vi "lorentzian transformations.vi"(7 "4 corner circle transformation":T3=enum."fix phase", 8 "lorentzian in":T2 {"bg (V)" format="%#9_9f"; "Q" format="%#9_9f"; "phi(rad)" format="%#9_9f"; "G (Hz)" format="%#9_9f"; "f (Hz)" format="%#9_9f"}, 10 "freq in":dbl, 11 "voltage in":cdb) -> (0 "lorentzian out":T2={"A (VHz)"=-1.0311345636926572, "f (Hz)"=-1.0311345636926572, "G (Hz)"=-1.0311345636926572, "phi(rad)"=-1.0311345636926572, "Q"=-1.0311345636926572, "Norm  Ampl"=-1.0311345636926572, "bg (V)"=-1.0311345636926572+0.0i, "4corners"={"z (-pi/2)"=-1.0311345636926572+0.5736824521422934i, "z(inf)"=-0.5200164984937075+1.0975277942502903i, "z (pi/2)"=-1.0311345636926572+0.5736824521422934i, "z center"=-0.5136528600391839+0.580046090596817i, "z(0)"=-0.5200164984937075+1.0975277942502903i, "radius"=-1.0311345636926572}} {"bg (V)" format="%#9_9f"; "Q" format="%#9_9f"; "phi(rad)" format="%#9_9f"; "G (Hz)" format="%#9_9f"; "f (Hz)" format="%#9_9f"}, 1 "4corners our":T1={"z (-pi/2)"=-1.0311345636926572+0.5736824521422934i, "z(inf)"=-0.5200164984937075+1.0975277942502903i, "z (pi/2)"=-1.0311345636926572+0.5736824521422934i, "z center"=-0.5136528600391839+0.580046090596817i, "z(0)"=-0.5200164984937075+1.0975277942502903i, "radius"=-1.0311345636926572}, 2 "gamma OUT":dbl, 3 "voltage out":cdb)   [LabVIEW 2018]
uses:
  four-corner circle transformation.ctl
  lorentzian.ctl
  circle corners.ctl
  Q - not nan -- real.vi
panel:
  out "freq OUT":dbl
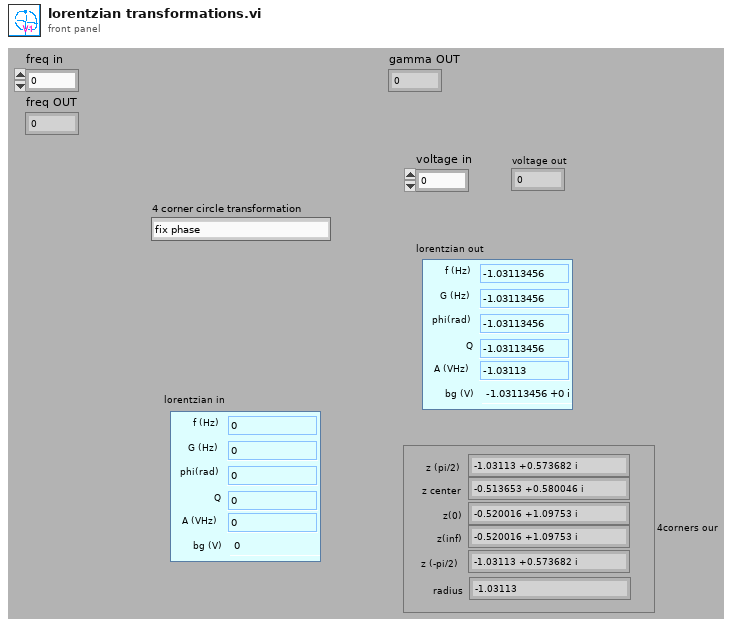
[diagram p1: front panel]
types:
  T1 = typedef "circle corners.ctl" = cluster{"z (-pi/2)":cdb, "z(inf)":cdb, "z (pi/2)":cdb, "z center":cdb, "z(0)":cdb, "radius":dbl}
  T2 = typedef "lorentzian.ctl" = cluster{"A (VHz)":dbl, "f (Hz)":dbl, "G (Hz)":dbl, "phi(rad)":dbl, "Q":dbl, "Norm  Ampl":dbl, "bg (V)":cdb, "4corners":T1}
  T3 = typedef "four-corner circle transformation.ctl" = enum16{"z(c) z(inf)", "z(c) z(zero)", "fix phase", "calculate lorentzian", "z(0) z(+-pi/2)", "shift to zcenter", "to  canonical", "get canonical phase", "get4corners", "update lorentzian -- from z0", "fake gamma normal", "fake gamma heat", "calculate complex slope"}
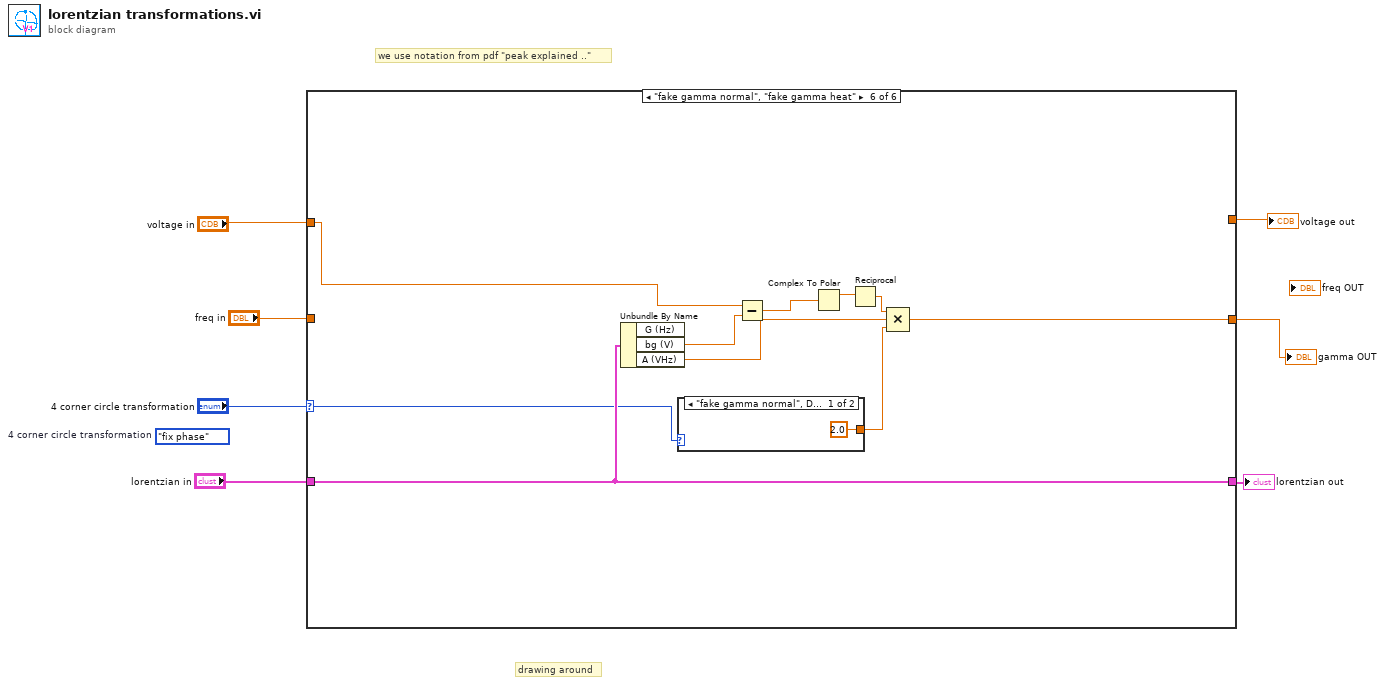
[diagram p0: block diagram]
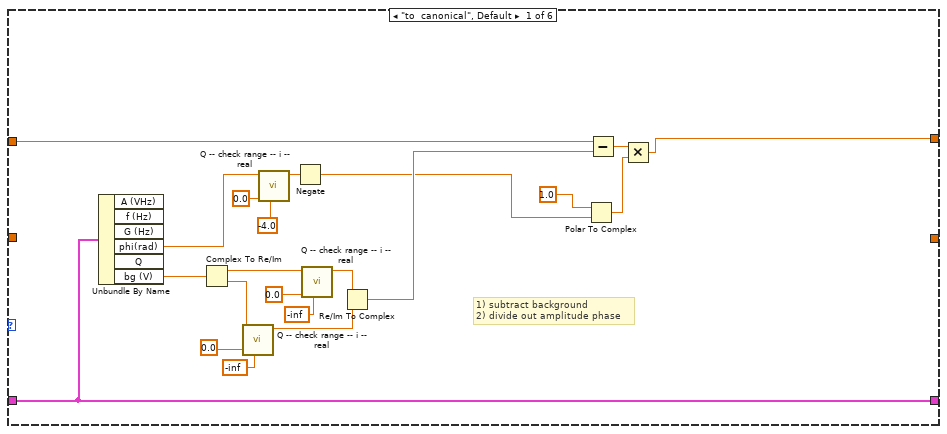
[diagram p2: hidden frame]
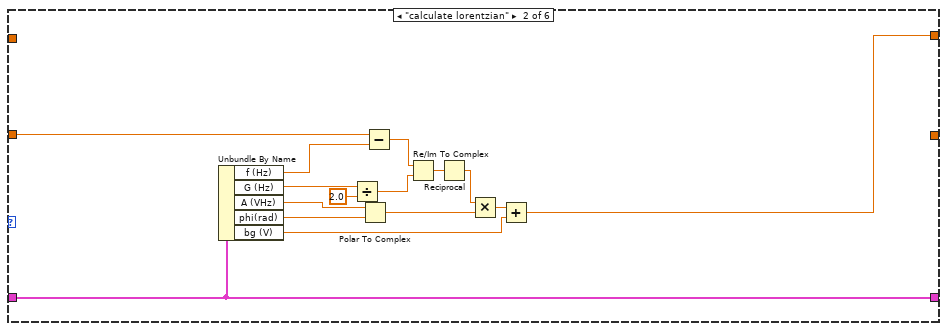
[diagram p3: hidden frame]
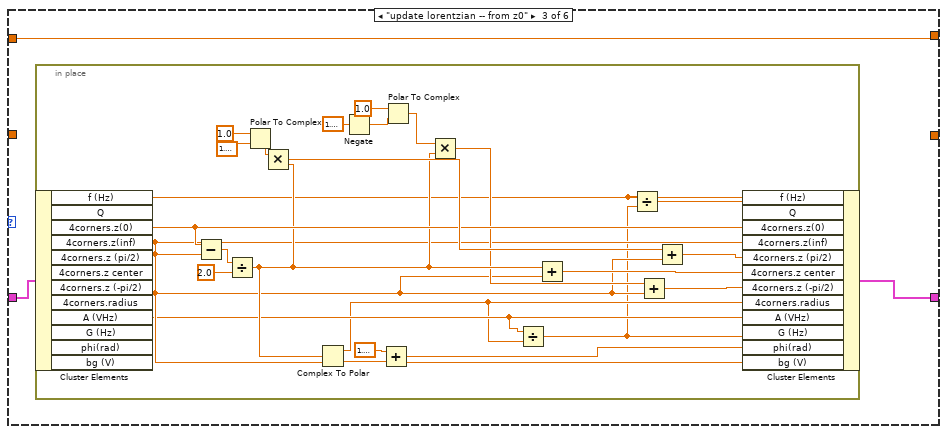
[diagram p4: hidden frame]
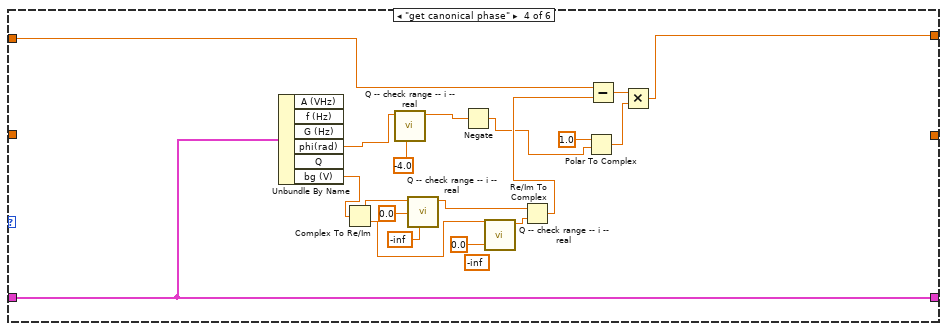
[diagram p5: hidden frame]
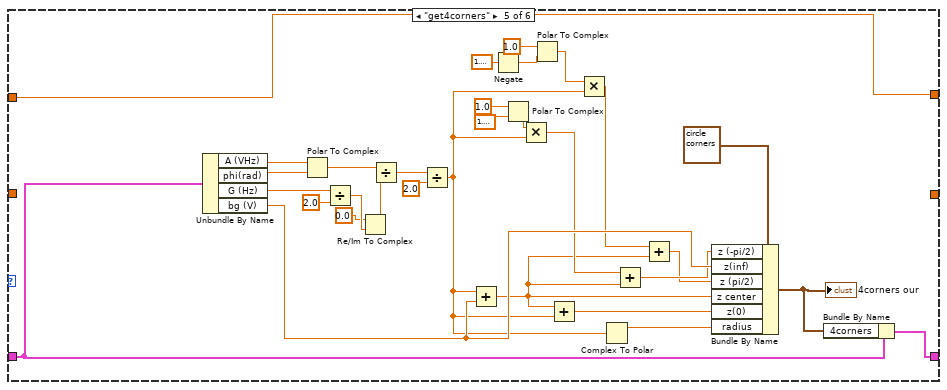
[diagram p6: hidden frame]
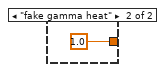
[diagram p7: hidden frame]
diagram:
  (unwired) four-corner_circle_transformation."fix phase"  # 4 corner circle transformation
  # "we use notation from pdf \"peak explained ..\""
  # "drawing around"
  n1 = case shown="\"fake gamma normal\", \"fake gamma heat\"" "4 corner circle transformation" {
    selector: "4 corner circle transformation" -> [_ _ _ _ _ w122]
    tunnel: "voltage in" -> [w11 _ w44 w73 w98 w125]
    tunnel: [w12 w43 w45 w74 w91 w124] -> w5
    tunnel: "lorentzian in" -> [w12 w43 w46 w74 w93 w124]
    tunnel: [w10 w37 w44 w72 w98 _] -> w3
    tunnel: "freq in" -> [_ w42 _ _ _ _]
    tunnel: [_ _ _ _ _ w123] -> w1
    frame "to  canonical", Default {
      # "1) subtract background\n2) divide out amplitude phase"
      n2 = Unbundle By Name(w12) -> ("phi(rad)"=w25:dbl, "bg (V)"=w23:cdb)  [unwired: 4 out]
      n3 = Complex To Re/Im(x + iy=w23) -> (x=w22:dbl, y=w20:dbl)
      n4 = call "Q -- check range -- i -- real.vi"("lower"=-inf, "default"=0.0, "number"=w20) -> ("number in range"=w17:dbl)  [unwired: 6 in, 2 out]
      n5 = call "Q -- check range -- i -- real.vi"("lower"=-4.0, "default"=0.0, "number"=w25) -> ("number in range"=w14:dbl)  [unwired: 6 in, 2 out]
      n6 = Negate(x=w14) -> (-x=w13:dbl)
      n7 = call "Q -- check range -- i -- real.vi"("lower"=-inf, "default"=0.0, "number"=w22) -> ("number in range"=w16:dbl)  [unwired: 6 in, 2 out]
      n8 = Re/Im To Complex(1:w17, 2:w16) -> (0:w15:cdb)
      n9 = Polar To Complex(1:w13, 2:1.0 ("r")) -> (0:w26:cdb)
      n10 = Subtract(x=w11, y=w15) -> (x-y=w27:cdb)
      n11 = Multiply(x=w27, y=w26) -> (x*y=w10:cdb)
    }
    frame "calculate lorentzian" {
      n12 = Unbundle By Name(w43) -> ("f (Hz)"=w30:dbl, "G (Hz)"=w29:dbl, "A (VHz)"=w31:dbl, "phi(rad)"=w41:dbl, "bg (V)"=w38:cdb)
      n13 = Divide(x=w29, y=2.0 ("x")) -> (x/y=w33:dbl)
      n14 = Polar To Complex(1:w41, 2:w31) -> (0:w40:cdb)
      n15 = Subtract(x=w42, y=w30) -> (x-y=w35:dbl)
      n16 = Re/Im To Complex(1:w33, 2:w35) -> (0:w32:cdb)
      n17 = Reciprocal(x=w32) -> (1/x=w36:cdb)
      n18 = Multiply(x=w36, y=w40) -> (x*y=w39:cdb)
      n19 = Add(x=w39, y=w38) -> (x+y=w37:cdb)
    }
    frame "update lorentzian -- from z0" {
      n20 = in-place {
        n21 = in-place-cluster #1(w46) -> ("f (Hz)"=w49:dbl, "4corners.z(0)"=w56:cdb, "4corners.z(inf)"=w52:cdb, "A (VHz)"=w51:dbl)  [unwired: 8 out]
        n22 = Subtract(x=w56, y=w52) -> (x-y=w67:cdb)
        n23 = Divide(x=w67, y=2.0) -> (x/y=w55:cdb)
        n24 = Polar To Complex(1:1.5707963267948966, 2:1.0 ("r")) -> (0:w60:cdb)
        n25 = Multiply(x=w60, y=w55) -> (x*y=w58:cdb)
        n26 = Complex To Polar(r * e^(i*theta)=w55) -> (r=w50:dbl, theta=w70:dbl)
        n27 = Negate(x=1.5707963267948966) -> (-x=w61:dbl)
        n28 = Add(x=1.5707963267948966, y=w70) -> (x+y=w69:dbl)
        n29 = Polar To Complex(1:w61, 2:1.0 ("r")) -> (0:w59:cdb)
        n30 = Multiply(x=w59, y=w55) -> (x*y=w54:cdb)
        n31 = Divide(x=w51, y=w50) -> (x/y=w48:dbl)
        n32 = Add(x=w55, y=w52) -> (x+y=w66:cdb)
        n33 = Divide(x=w49, y=w48) -> (x/y=w47:dbl)
        n34 = Add(x=w54, y=w52) -> (x+y=w53:cdb)
        n35 = Add(x=w58, y=w52) -> (x+y=w57:cdb)
        n36 = in-place-cluster #1("f (Hz)"=w49, "Q"=w47, "4corners.z(0)"=w56, "4corners.z(inf)"=w52, "4corners.z (pi/2)"=w57, "4corners.z center"=w66, "4corners.z (-pi/2)"=w53, "4corners.radius"=w50, "A (VHz)"=w51, "G (Hz)"=w48, "phi(rad)"=w69, "bg (V)"=w52) -> (w45:T2)
      }
    }
    frame "get canonical phase" {
      (unwired) -inf ("lower")
      n37 = Unbundle By Name(w74) -> ("phi(rad)"=w87:dbl, "bg (V)"=w85:cdb)  [unwired: 4 out]
      n38 = Complex To Re/Im(x + iy=w85) -> (x=w84:dbl, y=w82:dbl)
      n39 = call "Q -- check range -- i -- real.vi"("lower"=-4.0, "number"=w87) -> ("number in range"=w76:dbl)  [unwired: 7 in, 2 out]
      n40 = call "Q -- check range -- i -- real.vi"("lower"=-inf, "default"=0.0, "number"=w84) -> ("number in range"=w78:dbl)  [unwired: 6 in, 2 out]
      n41 = Negate(x=w76) -> (-x=w75:dbl)
      n42 = call "Q -- check range -- i -- real.vi"("default"=0.0, "number"=w82) -> ("number in range"=w79:dbl)  [unwired: 7 in, 2 out]
      n43 = Re/Im To Complex(1:w79, 2:w78) -> (0:w77:cdb)
      n44 = Polar To Complex(1:w75, 2:1.0 ("r")) -> (0:w88:cdb)
      n45 = Subtract(x=w73, y=w77) -> (x-y=w89:cdb)
      n46 = Multiply(x=w89, y=w88) -> (x*y=w72:cdb)
    }
    frame "get4corners" {
      n47 = Unbundle By Name(w93) -> ("A (VHz)"=w120:dbl, "phi(rad)"=w119:dbl, "G (Hz)"=w117:dbl, "bg (V)"=w106:cdb)
      n48 = Polar To Complex(1:w119, 2:w120) -> (0:w116:cdb)
      n49 = Divide(x=w117, y=2.0) -> (x/y=w101:dbl)
      n50 = Re/Im To Complex(1:w101, 2:0.0 ("x")) -> (0:w99:cdb)
      n51 = Divide(x=w116, y=w99) -> (x/y=w107:cdb)
      n52 = Divide(x=w107, y=2.0) -> (x/y=w94:cdb)
      n53 = Add(x=w94, y=w106) -> (x+y=w95:cdb)
      n54 = Negate(x=1.5707963267948966) -> (-x=w109:dbl)
      n55 = Polar To Complex(1:1.5707963267948966, 2:1.0 ("r")) -> (0:w105:cdb)
      n56 = Multiply(x=w105, y=w94) -> (x*y=w104:cdb)
      n57 = Polar To Complex(1:w109, 2:1.0 ("r")) -> (0:w103:cdb)
      n58 = Add(x=w95, y=w94) -> (x+y=w115:cdb)
      n59 = Multiply(x=w103, y=w94) -> (x*y=w102:cdb)
      n60 = Complex To Polar(r * e^(i*theta)=w94) -> (r=w114:dbl)  [unwired: 1 out]
      n61 = Add(x=w104, y=w95) -> (x+y=w97:cdb)
      n62 = Add(x=w102, y=w95) -> (x+y=w96:cdb)
      n63 = Bundle By Name(cluster=T1 {"z (-pi/2)"=-1.0311345636926572+0.5736824521422934i, "z(inf)"=-0.5200164984937075+1.0975277942502903i, "z (pi/2)"=-1.0311345636926572+0.5736824521422934i, "z center"=-0.5136528600391839+0.580046090596817i, "z(0)"=-0.5200164984937075+1.0975277942502903i, "radius"=-1.0311345636926572} ("circle corners"), "z (-pi/2)"=w97, "z(inf)"=w106, "z (pi/2)"=w96, "z center"=w95, "z(0)"=w115, "radius"=w114) -> (w92:T1)
      "4corners our" <- w92
      n64 = Bundle By Name(cluster=w93, "4corners"=w92) -> (w91:T2)
    }
    frame "fake gamma normal", "fake gamma heat" {
      n65 = Unbundle By Name(w124) -> ("bg (V)"=w127:cdb, "A (VHz)"=w126:dbl)  [unwired: 1 out]
      n66 = case shown="\"fake gamma normal\", Default" w122 {
        tunnel: [2.0 ("value") 1.0 ("value")] -> w131
        frame "fake gamma normal", Default {
        }
        frame "fake gamma heat" {
        }
      }
      n67 = Subtract(x=w125, y=w127) -> (x-y=w130:cdb)
      n68 = Complex To Polar(r * e^(i*theta)=w130) -> (r=w129:dbl)  [unwired: 1 out]
      n69 = Reciprocal(x=w129) -> (1/x=w128:dbl)
      n70 = Compound Arithmetic op=MULTIPLY(w128, w126, w131) -> (w123:dbl)
    }
  }
  "lorentzian out" <- w5
  "voltage out" <- w3
  "gamma OUT" <- w1
